vi "QP_Solver_pel.vi"(4 "equalityCons":bool[](array[boolean])=[FALSE, FALSE, FALSE, FALSE, FALSE, FALSE], 6 "DesiredFM":dbl[](array[numeric]), 7 "prevOP":dbl[](array[numeric]), 9 "Structural Matrix":dbl[][](array[numeric]), 11 "Constants HL":T1={"Frame Points"=[], "Brace Points in P"=[], "QP_lb"=[], "QP_ub"=[], "Q for QP"=[], "nMotors"=0, "QP stopping criteria"={"function tolerance"=1e-08, "parameter tolerance"=1000000.0, "max iterations"=10000, "max function calls"=10000, "gradient tolerance"=1000000.0, "max time (sec)"=-1.0}, "MotorsPos_wrt_Markers"=[], "nMotors 1"=0, "nMotors 2"=0, "MotorsPos_wrt_Markers pel"=[], "Frame Points_pel"=[], "Brace Points in P_pel"=[], "QP_lb pel"=[], "QP_ub pel"=[], "Q for QP pel"=[], "MotorsPos_wrt_Markers knees"=[], "nMotors 3"=0}) -> (0 "error out":errorcluster, 2 "scaledT":dbl[](array[numeric]), 3 "min T":dbl[](array[numeric]))   [LabVIEW 2017]
uses:
  typeDef/constants_HL.ctl
  <vilib>/gmath/NumericalOptimization/stopping criteria.ctl
  <vilib>/imath/engines/lvmath2/RunTimeEngine/RangeToken/NIMS_Range_R2 - Integer.vi
  <instcachedir>/0/NIMS_Range_R2 - Integer_B2C3C6B11D0E4F789E1772ACB483EB02.lvgen/NIMS_Range_R2 - Integer_B2C3C6B11D0E4F789E1772ACB483EB02_000.vi
  <vilib>/imath/engines/lvmath2/RunTimeEngine/CommandStatement/MC_CommandStatement_break.vi
  <vilib>/imath/engines/lvmath2/RunTimeEngine/IndexRead/NIMS V(S).vi
  <instcachedir>/0/NIMS V(S)_0488751826AF41519A22953C041130DC.lvgen/NIMS V(S)_0488751826AF41519A22953C041130DC_003.vi
  <vilib>/imathl/engines/lvmath/Functions/Error Handling/Create Error.vi
  <vilib>/imath/engines/lvmath2/RunTimeEngine/VariableToken/NIMS_VariableToken_CondDefinedDefinedByReplace.vi
  <instcachedir>/0/NIMS_VariableToken_CondDefinedDefinedByReplace_D162CFFC24174562A9FEA619A91E1A56.lvgen/NIMS_VariableToken_CondDefinedDefinedByReplace_D162CFFC24174562A9FEA619A91E1A56_001.vi
  <vilib>/imath/engines/lvmath2/RunTimeEngine/IndexRead/NIMS M(S,$).vi
  <instcachedir>/0/NIMS M(S,$)_F24F360562DE41D8BE234322A2E15C65.lvgen/NIMS M(S,$)_F24F360562DE41D8BE234322A2E15C65_000.vi
  <vilib>/imath/engines/lvmath2/RunTimeEngine/IndexReplace/NIMS M(S,R2)=V.vi
  <instcachedir>/0/NIMS M(S,R2)=V_7A6CBA24A40E4522B17742971865BE90.lvgen/NIMS M(S,R2)=V_7A6CBA24A40E4522B17742971865BE90_000.vi
  <vilib>/imath/engines/lvmath2/RunTimeEngine/ErrorHandling/NIMS_Create Error From Enums.vi
  <instcachedir>/0/NIMS_VariableToken_CondDefinedDefinedByReplace_D162CFFC24174562A9FEA619A91E1A56.lvgen/NIMS_VariableToken_CondDefinedDefinedByReplace_D162CFFC24174562A9FEA619A91E1A56_002.vi
  <instcachedir>/0/NIMS V(S)_0488751826AF41519A22953C041130DC.lvgen/NIMS V(S)_0488751826AF41519A22953C041130DC_000.vi
  <vilib>/imath/engines/lvmath2/RunTimeEngine/IndexReplace/NIMS V(S)=S.vi
  <instcachedir>/0/NIMS V(S)=S_3F4D177D41884A9C969E5FA0B22E4B28.lvgen/NIMS V(S)=S_3F4D177D41884A9C969E5FA0B22E4B28_000.vi
  <vilib>/imath/engines/lvmath2/RunTimeEngine/VariableToken/NIMS_VariableToken_CondDefined.vi
  <instcachedir>/0/NIMS_VariableToken_CondDefined_6E7F1EE7F80E48298C84CF05BD736261.lvgen/NIMS_VariableToken_CondDefined_6E7F1EE7F80E48298C84CF05BD736261_001.vi
  <instcachedir>/0/NIMS_VariableToken_CondDefined_6E7F1EE7F80E48298C84CF05BD736261.lvgen/NIMS_VariableToken_CondDefined_6E7F1EE7F80E48298C84CF05BD736261_003.vi
  <vilib>/imath/engines/lvmath/Functions/Error Handling/MergeErrorsWrapper.vi
  <vilib>/imath/engines/lvmath2/RunTimeEngine/NodeEndStatement/NIMS_NodeEndStatement_Output.vi
  <instcachedir>/0/NIMS_NodeEndStatement_Output_53EC0D466D134D7ABD903AC30B43404B.lvgen/NIMS_NodeEndStatement_Output_53EC0D466D134D7ABD903AC30B43404B_005.vi
  <instcachedir>/0/NIMS_NodeEndStatement_Output_53EC0D466D134D7ABD903AC30B43404B.lvgen/NIMS_NodeEndStatement_Output_53EC0D466D134D7ABD903AC30B43404B_002.vi
  <vilib>/imath/engines/lvmath2/RunTimeEngine/ErrorHandling/NIMS_Finalize Error.vi
  <vilib>/gmath/NumericalOptimization/Quadratic Programming AS.vi
  <vilib>/gmath/NI_Gmath.lvlib
panel:
  in  "Q for QP pel -scaled":dbl[][](array[numeric])=[[1.5, 0.0, 0.0, 0.0, 0.0, 0.0, 0.0, 0.0], [0.0, 1.5, 0.0, 0.0, 0.0, 0.0, 0.0, 0.0], [0.0, 0.0, 1.0, 0.0, 0.0, 0.0, 0.0, 0.0], [0.0, 0.0, 0.0, 1.0, 0.0, 0.0, 0.0, 0.0], [0.0, 0.0, 0.0, 0.0, 1.5, 0.0, 0.0, 0.0], [0.0, 0.0, 0.0, 0.0, 0.0, 1.5, 0.0, 0.0], [0.0, 0.0, 0.0, 0.0, 0.0, 0.0, 1.0, 0.0], [0.0, 0.0, 0.0, 0.0, 0.0, 0.0, 0.0, 1.0]]
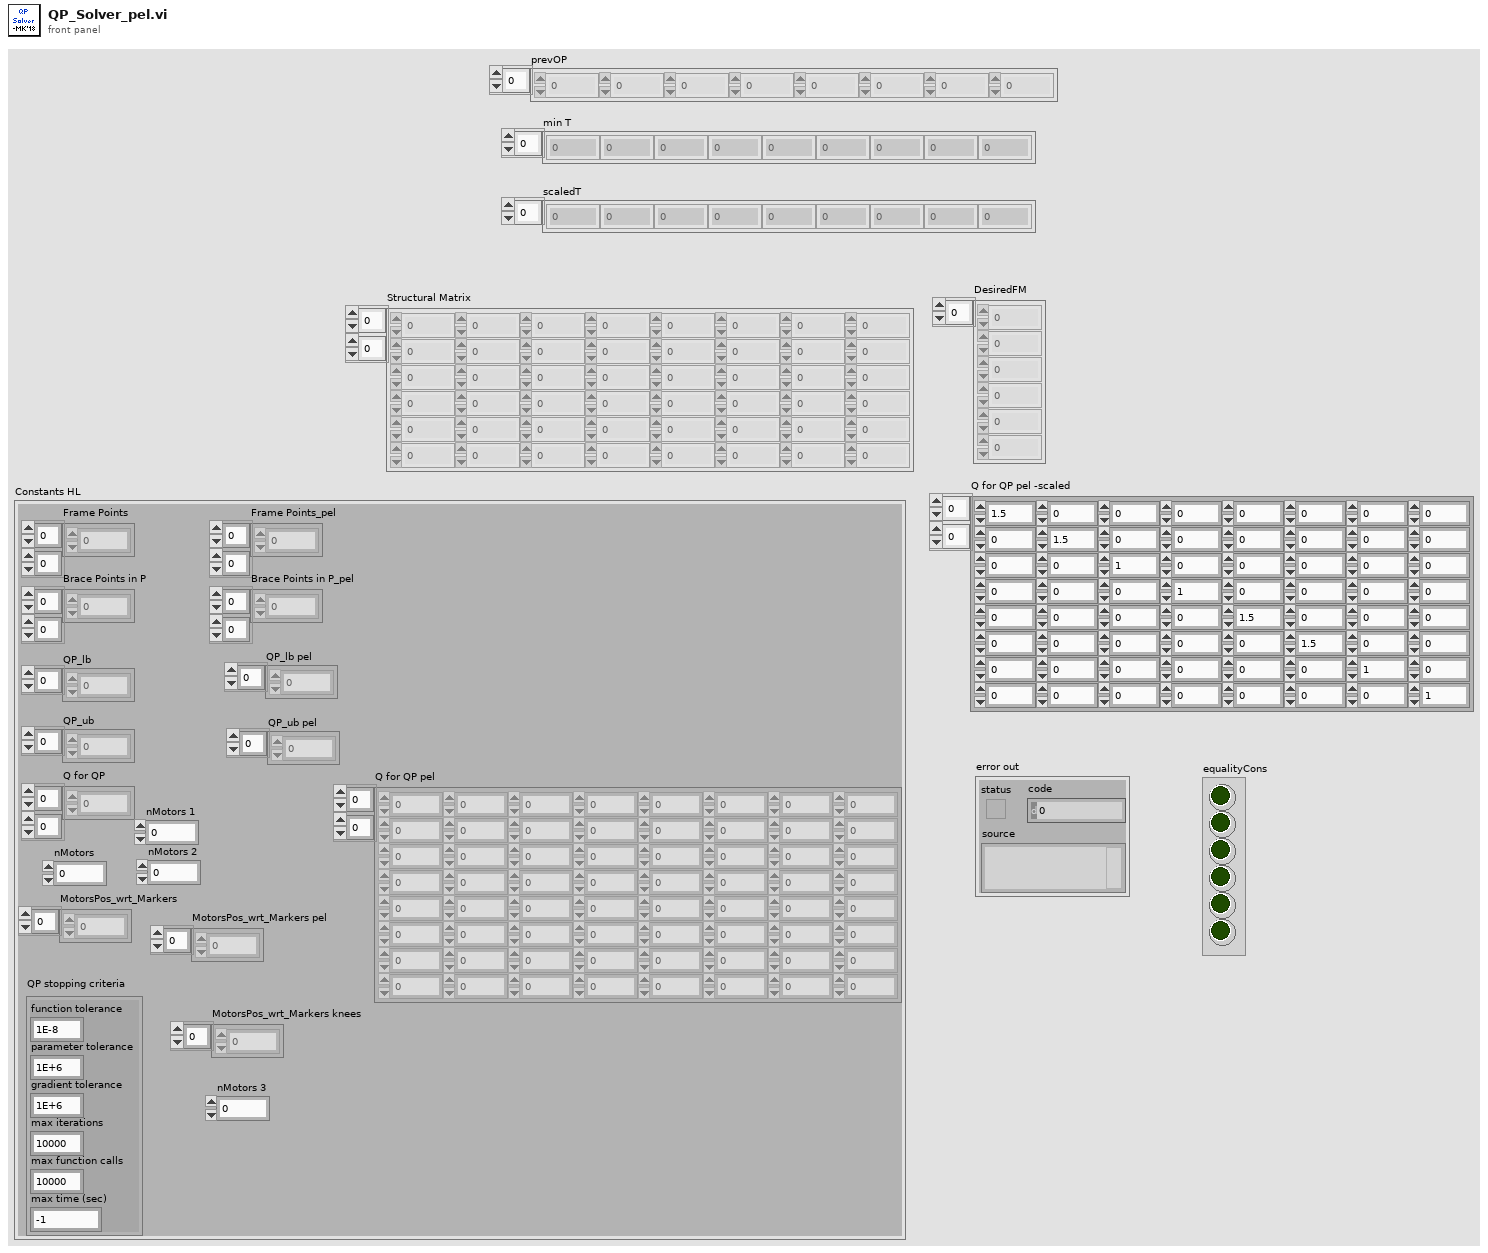
[diagram p1: front panel]
types:
  T1 = typedef "constants_HL.ctl" = cluster{"Frame Points":dbl[][], "Brace Points in P":dbl[][], "QP_lb":dbl[], "QP_ub":dbl[], "Q for QP":dbl[][], "nMotors":i32, "QP stopping criteria":T2, "MotorsPos_wrt_Markers":i32[], "nMotors 1":i32, "nMotors 2":i32, "MotorsPos_wrt_Markers pel":i32[], "Frame Points_pel":dbl[][], "Brace Points in P_pel":dbl[][], "QP_lb pel":dbl[], "QP_ub pel":dbl[], "Q for QP pel":dbl[][], "MotorsPos_wrt_Markers knees":i32[], "nMotors 3":i32}
  T2 = typedef "NI_Gmath.lvlib/stopping criteria.ctl" = cluster{"function tolerance":dbl, "parameter tolerance":dbl, "max iterations":i32, "max function calls":i32, "gradient tolerance":dbl, "max time (sec)":dbl}
  T3 = cluster{"Aieq":dbl[][], "Imin":dbl[], "Imax":dbl[]}
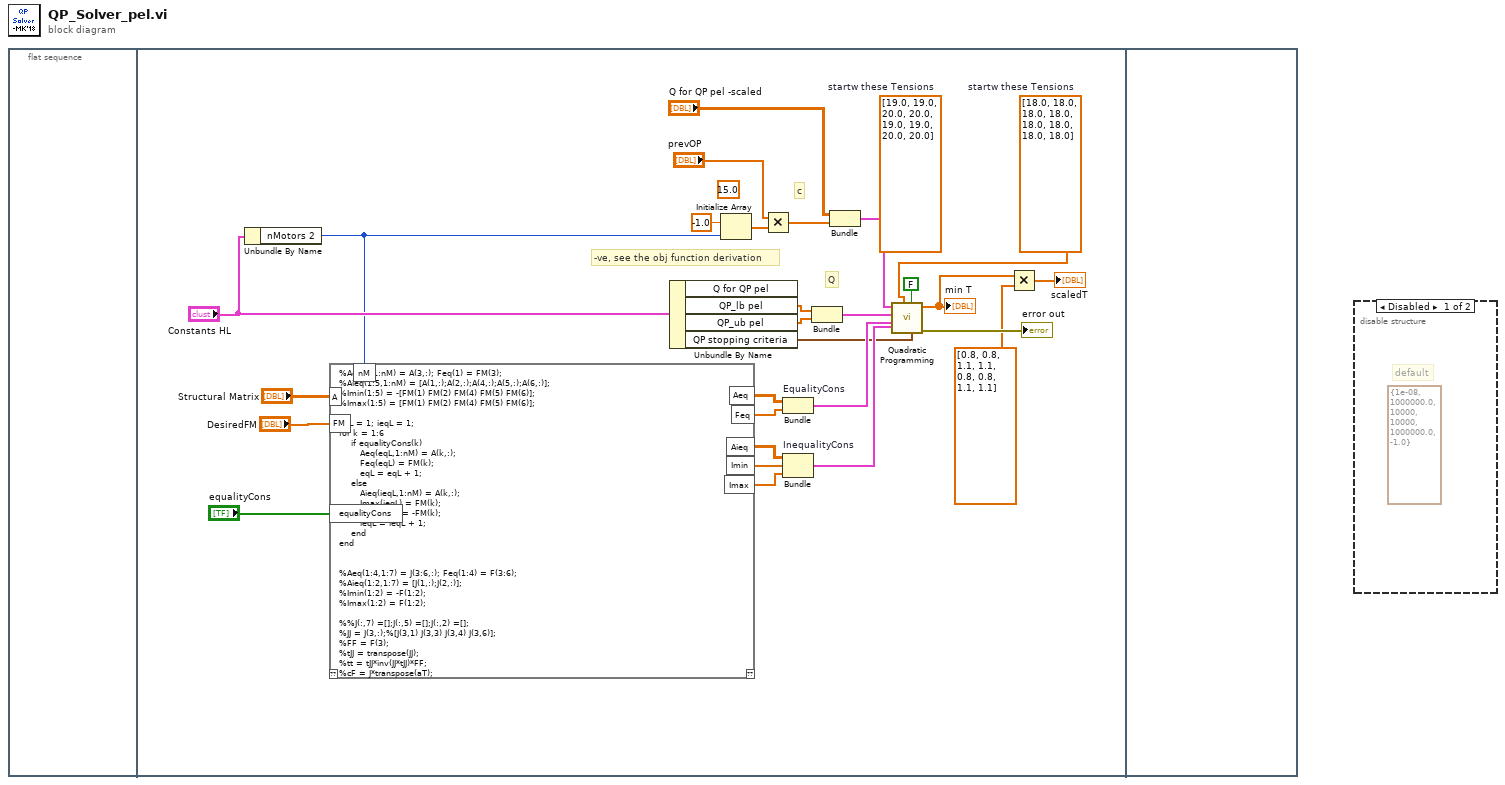
[diagram p0: block diagram]
diagram:
  n1 = flat-sequence {
    frame #0 {
    }
    frame #1 {
      w1 = dbl[] [18.0, 18.0, 18.0, 18.0, 18.0, 18.0, 18.0, 18.0]  # startw these Tensions
      (unwired) dbl[] [19.0, 19.0, 20.0, 20.0, 19.0, 19.0, 20.0, 20.0]  # startw these Tensions
      (unwired) 15.0 ("element")
      # "c"
      # "Q"
      # "-ve, see the obj function derivation"
      n2 = Unbundle By Name("Constants HL") -> ("nMotors 2"=w9:i32)
      n3 = mathscript code="%Aeq(1,1:nM) = A(3,:); Feq(1) = FM(3);\n%Aieq(1:5,1:nM) = [A(1,:);A(2,:);A(4,:);A(5,:);A(6,:)];\n%Imin(1:5) = -[FM(1) FM(2) FM(4) FM(5) FM(6)];\n%Imax(1:5) = [FM(1) FM(2) FM(4) FM(5) FM(6)];\n\neqL = 1; ieqL = 1;\nfor k = 1:6\n    if equalityCons(k)\n       Aeq(eqL,1:nM) = A(k,:);\n       Feq(eqL) = FM(k);\n       eqL = eqL + 1;\n    else\n       Aieq(ieqL,1:nM) = A(k,:);\n       Imax(ieqL) = FM(k);\n       Imin(ieqL) = -FM(k);\n       ieqL = ieqL + 1;\n    end\nend\n\n\n%Aeq(1:4,1:7) = J(3:6,:); Feq(1:4) = F(3:6);\n%Aieq(1:2,1:7) = [J(1,:);J(2,:)];\n%Imin(1:2) = -F(1:2);\n%Imax(1:2) = F(1:2);\n\n%%J(:,7) =[];J(:,5) =[];J(:,2) =[];\n%JJ = J(3,:);%[J(3,1) J(3,3) J(3,4) J(3,6)];\n%FF = F(3);\n%tJJ = transpose(JJ);\n%tt = tJJ*inv(JJ*tJJ)*FF;\n%cF = J*transpose(aT);"("A"="Structural Matrix", "FM"="DesiredFM", "nM"=w9, "equalityCons"="equalityCons") -> ("Aeq"=w23:dbl[][], "Feq"=w22:dbl[], "Aieq"=w21:dbl[][], "Imin"=w20:dbl[], "Imax"=w19:dbl[])  [unwired: 1 in, 1 out]
      n4 = Unbundle By Name("Constants HL") -> ("QP_lb pel"=w13:dbl[], "QP_ub pel"=w14:dbl[], "QP stopping criteria"=w8:T2)  [unwired: 1 out]
      n5 = Initialize Array(-1.0 ("element"), w9) -> (w26:dbl[])
      n6 = Multiply(x="prevOP", y=w26) -> (x*y=w28:dbl[])
      n7 = Bundle "EqualityCons"("Aeq"=w23, "Feq"=w22) -> (w18:cluster{"Aeq":dbl[][], "Feq":dbl[]})  [unwired: 1 in]
      n8 = Bundle "InequalityCons"("Aieq"=w21, "Imin"=w20, "Imax"=w19) -> (w17:T3)  [unwired: 1 in]
      n9 = Bundle("QP_lb pel"=w13, "QP_ub pel"=w14) -> (w12:cluster{"QP_lb pel":dbl[], "QP_ub pel":dbl[]})  [unwired: 1 in]
      n10 = Bundle("Q for QP pel -scaled"="Q for QP pel -scaled", w28) -> (w24:cluster{"Q for QP pel -scaled":dbl[][], dbl[]})  [unwired: 1 in]
      n11 = call-poly <vilib>:"Quadratic Programming.vi"("stopping criteria"=w8, "warm start?"=FALSE, "inequality constraints"=w17, "start"=w1, "equality constraints"=w18, "parameter bounds"=w12, "objective function"=w24) -> ("error out"=→"error out":errorcluster, "minimum"=w6:dbl[])  [unwired: 1 in, 2 out]
      "min T" <- w6
      n12 = Multiply(x=w6, y=dbl[] [0.8, 0.8, 1.1, 1.1, 0.8, 0.8, 1.1, 1.1] ("array")) -> (x*y=→"scaledT":dbl[])
    }
    frame #2 {
    }
  }
  n13 = disable-structure shown="Disabled" {
    frame Disabled {
      (unwired) T2 {"function tolerance"=1e-08, "parameter tolerance"=1000000.0, "max iterations"=10000, "max function calls"=10000, "gradient tolerance"=1000000.0, "max time (sec)"=-1.0} ("stopping criteria")
      # "default"
    }
    frame Enabled {
    }
  }
